vi "Move the EXE.vi"(0 "Primary destination path":path, 11 "error in (no error)":errorcluster) -> (15 "error out":errorcluster)   [LabVIEW 2021, in "Packager Helpers.lvlib"]
uses:
  Packager Helpers.lvlib
  Path Functions/Path Functions.lvlib
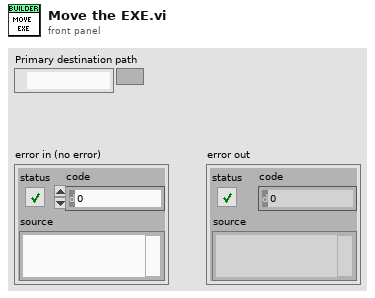
[diagram p1: front panel]
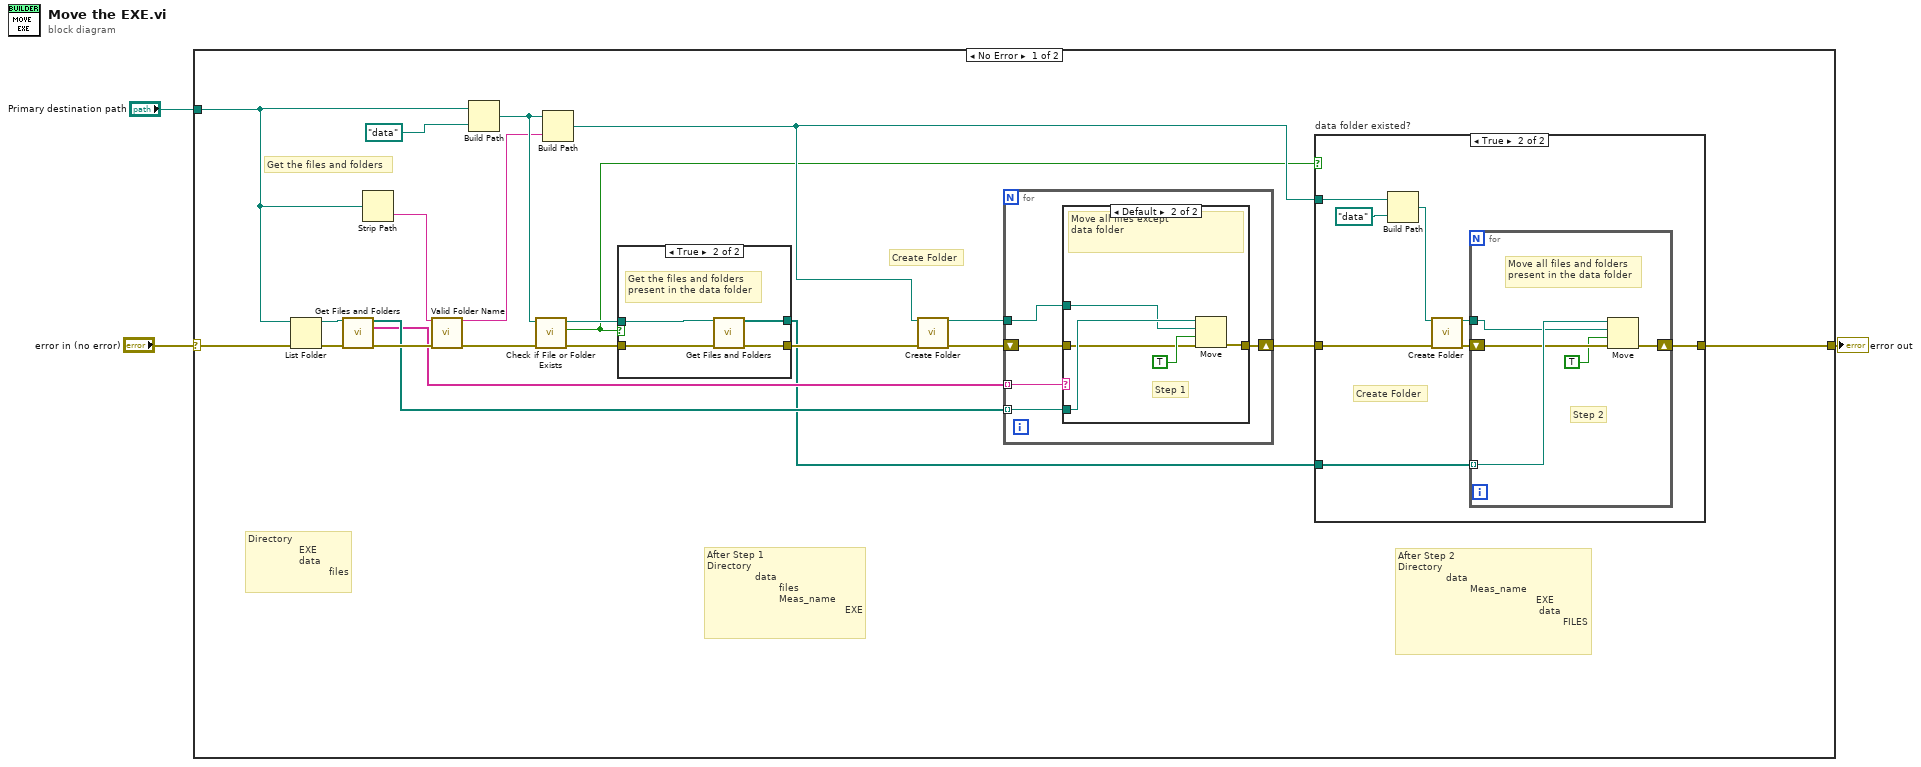
[diagram p0: block diagram]
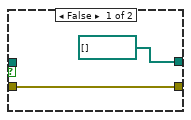
[diagram p3: hidden frame]
diagram:
  n1 = case shown="No Error" "error in (no error)" {
    selector: "error in (no error)" -> [w25 w57]
    tunnel: "Primary destination path" -> [w23 _]
    tunnel: [w5 w57] -> w1
    frame No Error {
      # "Directory\n                 EXE\n                 data\n                           files"
      # "Create Folder"
      # "Get the files and folders"
      # "After Step 2\nDirectory\n                data\n                        Meas_name\n                                              EXE\n                                               data\n                                                       FILES"
      # "After Step 1\nDirectory\n                data\n                        files\n                        Meas_name\n                                              EXE"
      n2 = List Folder(path=w23, error in=w25) -> (path out=w19:path, error out=w18:errorcluster)  [unwired: 2 in, 2 out]
      n3 = call "Get Files and Folders.vi"("File Directory"=w19, "error in (no error)"=w18) -> ("Files and Folders"=w12:path[], "Files and Folder Names"=w9:string[], "error out"=w14:errorcluster)  [unwired: 11 in]
      n4 = Strip Path(path=w23) -> (name=w17:string)  [unwired: 1 out]
      n5 = call "Valid Folder Name.vi"("Package"=w17, "error in (no error)"=w14) -> ("Valid Package Name"=w16:string, "error out"=w15:errorcluster)  [unwired: 12 in]
      n6 = Build Path(base path=w23, name or relative path=path "data") -> (appended path=w22:path)
      n7 = call <vilib>:"Check if File or Folder Exists.vi"("error in (no error)"=w15, "path"=w22) -> ("error out"=w20:errorcluster, "file or folder exists?"=w4:bool, "dup path"=w21:path)  [unwired: 7 in]
      n8 = Build Path(base path=w22, name or relative path=w16) -> (appended path=w8:path)
      n9 = case shown="True" w4 {
        tunnel: w21 -> [_ w40]
        tunnel: w20 -> [w38 w42]
        tunnel: [w38 w41] -> w13
        tunnel: [path[] [] ("Files and Folders") w39] -> w6
        frame False {
        }
        frame True {
          # "Get the files and folders\npresent in the data folder"
          n10 = call "Get Files and Folders.vi"("File Directory"=w40, "error in (no error)"=w42) -> ("Files and Folders"=w39:path[], "error out"=w41:errorcluster)  [unwired: 11 in, 1 out]
        }
      }
      n11 = call "Create Folder.vi"("Directory Path"=w8, "error in (no error)"=w13) -> ("Dup Directory Path"=w11:path, "error out"=w10:errorcluster)  [unwired: 12 in]
      n12 = for {
        tunnel: w12 -> [w30] mode=indexing
        tunnel: w11 -> [w29]
        shift-right: [w26] -> w7
        shift-left: w10 -> [w28]
        tunnel: w9 -> [w27] mode=indexing
        n13 = case shown="Default" w27 {
          tunnel: w30 -> [_ w36]
          tunnel: w29 -> [_ w35]
          tunnel: w28 -> [w31 w33]
          tunnel: [w31 w32] -> w26
          frame "data" {
          }
          frame Default {
            # "Step 1"
            # "Move all files except\ndata folder"
            n14 = Move(source path=w36, error in=w33, 9:TRUE ("overwrite (F)"), 10:w35) -> (error out=w32:errorcluster)  [unwired: 1 in, 2 out]
          }
        }
      }
      n15 = case "data folder existed?" shown="True" w4 {
        tunnel: w8 -> [_ w51]
        tunnel: w7 -> [w43 w48]
        tunnel: w6 -> [_ w46]
        tunnel: [w43 w44] -> w5
        frame False {
        }
        frame True {
          # "Create Folder"
          n16 = Build Path(base path=w51, name or relative path=path "data") -> (appended path=w49:path)
          n17 = call "Create Folder.vi"("Directory Path"=w49, "error in (no error)"=w48) -> ("Dup Directory Path"=w47:path, "error out"=w45:errorcluster)  [unwired: 12 in]
          n18 = for {
            tunnel: w46 -> [w56] mode=indexing
            tunnel: w47 -> [w55]
            shift-right: [w53] -> w44
            shift-left: w45 -> [w54]
            # "Move all files and folders\npresent in the data folder"
            # "Step 2"
            n19 = Move(source path=w56, error in=w54, 9:TRUE ("overwrite (F)"), 10:w55) -> (error out=w53:errorcluster)  [unwired: 1 in, 2 out]
          }
        }
      }
    }
    frame Error {
    }
  }
  "error out" <- w1
